vi "IfFoldExistDeleteThenCreatNewFold.vi"(1 "FoldPath in":path=path "C:/Users/tina_lai/Desktop/cap/PCBModel/PCBModel_002/fabmastr.txt") -> (0 "FoldPath out":path=path "C:/Users/tina_lai/Desktop/cap/PCBModel/PCBModel_002/fabmastr.txt")   [LabVIEW 2014]
panel:
  out "error out":errorcluster
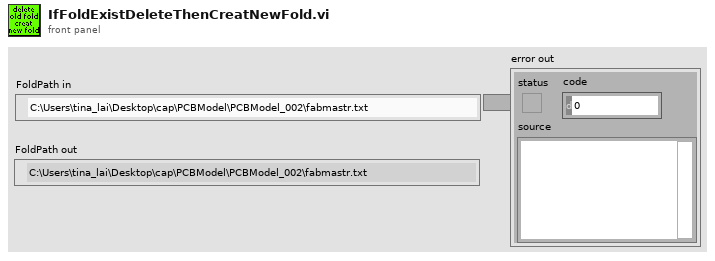
[diagram p1: front panel]
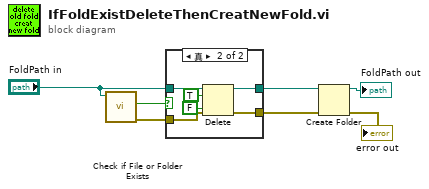
[diagram p0: block diagram]
diagram:
  n1 = call <vilib>:"Check if File or Folder Exists.vi"("path"="FoldPath in") -> ("error out"=w2:errorcluster, "file or folder exists?"=w6:bool)  [unwired: 8 in, 1 out]
  n2 = case shown="真" w6 {
    tunnel: "FoldPath in" -> [w9 w15]
    tunnel: [w9 w13] -> w5
    tunnel: [w8 w12] -> w3
    tunnel: w2 -> [w8 w11]
    frame False {
    }
    frame True {
      n3 = Delete(path (use dialog)=w15, entire hierarchy (F)=TRUE, confirm (F)=FALSE, error in=w11) -> (deleted path=w13:path, error out=w12:errorcluster)  [unwired: 1 in, 1 out]
    }
  }
  n4 = Create Folder(path (use dialog)=w5, error in=w3) -> (created path=→"FoldPath out":path, error out=→"error out":errorcluster)  [unwired: 1 in, 1 out]
